vi "LEBITplc.ParseScale&OffsetArray.vi"(2 "ScaleAndOffsetArray":string[][](array[string])) -> (14 "ScaleServicesID":i32[](array[numeric]), 16 "OffsetServicesID":i32[](array[numeric]), 17 "AllPLCValues":string[](array[string]), 18 "Scale":dbl[](array[numeric]), 19 "Offset":dbl[](array[numeric]))   [LabVIEW 2014, in "LEBITplc.lvlib"]
uses:
  LEBITplc.lvlib
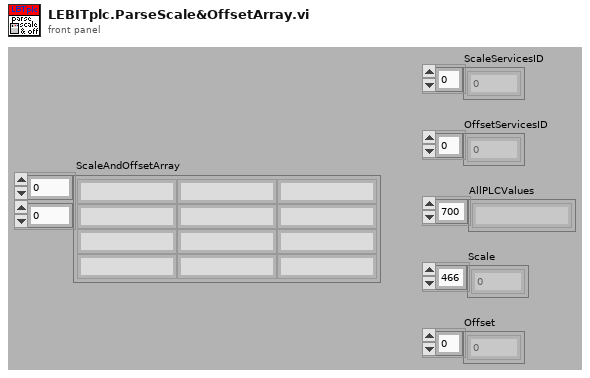
[diagram p1: front panel]
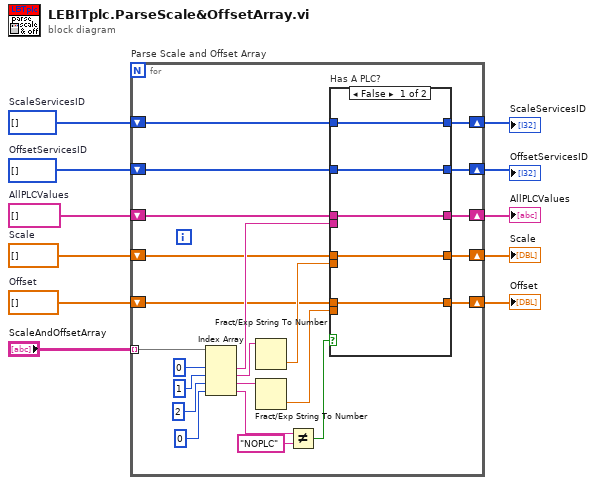
[diagram p0: block diagram]
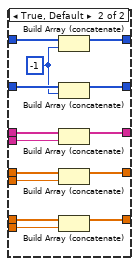
[diagram p2: hidden frame]
diagram:
  w9 = string[] []  # AllPLCValues
  w3 = i32[] []  # OffsetServicesID
  w1 = i32[] []  # ScaleServicesID
  w10 = dbl[] []  # Offset
  w11 = dbl[] []  # Scale
  n1 = for "Parse Scale and Offset Array" {
    tunnel: "ScaleAndOffsetArray" -> [w32] mode=indexing
    shift-right: [w22] -> w6
    shift-left: w9 -> [w19]
    shift-right: [w21] -> w8
    shift-left: w3 -> [w33]
    shift-right: [w20] -> w7
    shift-left: w1 -> [w34]
    shift-right: [w25] -> w4
    shift-left: w11 -> [w17]
    shift-right: [w16] -> w5
    shift-left: w10 -> [w18]
    n2 = Index Array(array=w32, index #1=0 ("index"), index #2=1 ("disabled index (row)"), index #3=2 ("index"), index #4=0 ("index")) -> (element #1=w26:string, element #2=w28:string, element #3=w27:string, element #4=w13:string)
    n3 = Fract/Exp String To Number(string=w28) -> (number=w24:dbl)  [unwired: 3 in, 1 out]
    n4 = Fract/Exp String To Number(string=w27) -> (number=w23:dbl)  [unwired: 3 in, 1 out]
    n5 = Not Equal?(x=w13, y="NOPLC") -> (x != y?=w12:bool)
    n6 = case "Has A PLC?" shown="False" w12 {
      tunnel: w34 -> [w39 w53]
      tunnel: w33 -> [w38 w52]
      tunnel: w26 -> [_ w50]
      tunnel: [w36 w49] -> w25
      tunnel: w24 -> [_ w48]
      tunnel: w23 -> [_ w47]
      tunnel: [w37 w46] -> w22
      tunnel: [w38 w45] -> w21
      tunnel: [w39 w44] -> w20
      tunnel: w19 -> [w37 w43]
      tunnel: w18 -> [w35 w42]
      tunnel: w17 -> [w36 w41]
      tunnel: [w35 w40] -> w16
      frame False {
      }
      frame True, Default {
        w51 = -1
        n7 = Build Array (concatenate)(w53, w51) -> (w44:i32[])
        n8 = Build Array (concatenate)(w52, w51) -> (w45:i32[])
        n9 = Build Array (concatenate)(w43, w50) -> (w46:string[])
        n10 = Build Array (concatenate)(w41, w48) -> (w49:dbl[])
        n11 = Build Array (concatenate)(w42, w47) -> (w40:dbl[])
      }
    }
  }
  "ScaleServicesID" <- w7
  "Scale" <- w4
  "Offset" <- w5
  "OffsetServicesID" <- w8
  "AllPLCValues" <- w6
